vi "CC Script GUI.vi"(10 "Standalone":bool=TRUE, 11 "Cmd Qs":T1) -> ()   [LabVIEW 2024]
uses:
  Subsystems/SS cluster Command Queues.ctl
  Subsystems/SS typedef Cmd Queue Reference.ctl
  Subsystems/SS typedef cluster Instrument Command Queue Data.ctl
  CC cluster Script Panel Defaults.ctl
  typedefs/CC Script Step.ctl
  typedefs/CC enum Script Action.ctl
  typedefs/CC cluster Exposure.ctl
  Detector/Detector Class/Detector enum Detector Integration Mode.ctl
  typedefs/CC cluster Object.ctl
  typedefs/CC cluster sidereal rate.ctl
  typedefs/CC cluster RA and DEC.ctl
  typedefs/cc cluster muRA muDEC.ctl
  Telescope/CC cluster Telescope Offsets.ctl
  typedefs/CC cluster Acquire Parameters.ctl
  Subsystems/SS cluster Script Status Queue.ctl
  typedefs/CC cluster Random Dithering.ctl
  typedefs/CC Dithering.ctl
  typedefs/CC cluster Offset Dithering.ctl
  typedefs/CC Dithering Offsets.ctl
  typedefs/CC cluster Observation Record.ctl
  Subsystems/SS cluster New Image Data.ctl
  hk-channel-class/hk-channel-class/HK Item/HK Item.lvclass
  Subsystems/SS cluster Data Queue type.ctl
  typedefs/CC cluster Observation.ctl
  Observation Queue/CC enum Observation Status.ctl
  typedefs/CC cluster Observation Dither Options.ctl
  typedefs/CC enum Dither Selection.ctl
  typedefs/CC cluster Script.ctl
  typedefs/CC cluster Script Status Data.ctl
  typedefs/CC cluster Pause Parameters.ctl
  Filter Wheel/FW cmd Q Move Parameters.ctl
  Logging/CC enum Current Values Action.ctl
  Focus/Focus cluster MoveFocus Command Parameters.ctl
  CC Rd Wr Script Action.ctl
  3a551b90-7109-44fc-bb48-53d4c8d7d9ea.vi
  fb980131-14b8-4ba4-a5ba-d8795c8df878.vi
  73e8f019-b90d-454d-a375-f578a22e9470.vi
  6180e3d0-9506-4a5f-afbf-da5a1e2ce68c.vi
  79eba822-2b6b-4a1a-8f0f-f154aabb2b36.vi
  hk-channel-class/hk-channel-class/HK Table/HK Table.lvclass
  <vilib>/Utility/Data Type/NI_Data Type.lvlib
panel:
  in  "Script Path":path
  in  "Pause Button":bool
  out "Running":bool
  in  "Close":bool
  in  "Stop Script":bool
  in  "New Script":bool
  in  "Edit Script":bool
  in  "Run Script":bool
  in  "Script":string(combo)
  in  "Script":i32(listbox)
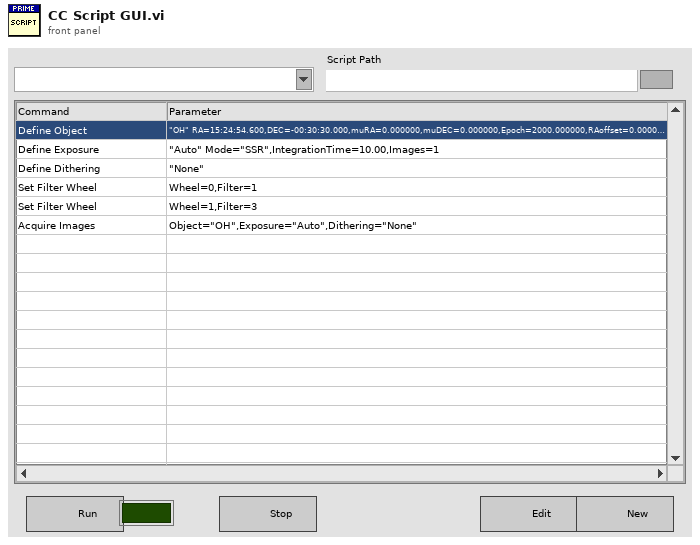
[diagram p1: front panel]
types:
  T1 = typedef "SS cluster Command Queues.ctl" = cluster{"Telescope Q":T2, "Filter Wheel Q":T2, "Script Q":T2, "CryoServer Q":T2, "Detector Q":T2, "Focus Q":T2}
  T2 = typedef "SS typedef Cmd Queue Reference.ctl" = refnum<queue>
  T3 = typedef "CC cluster Script Panel Defaults.ctl" = cluster{"Script Name":string, "Script Path":path}
  T4 = typedef "CC Script Step.ctl" = cluster{"Action":T5, "Data":variant}
  T5 = typedef "CC enum Script Action.ctl" = enum16{"Noop", "Define Object", "Define Exposure", "Define Dithering", "Acquire Images", "Set Filter Wheel", "Telescope Home", "Telescope Move", "Telescope RA DEC", "Focus Move Relative", "Focus Move Absolute", "Focus Set Home", "Macro", "Pause", "Ask User", "Define Random Dither"}
  T6 = typedef "CC cluster Exposure.ctl" = cluster{"Mode":T7, "Integration Time":dbl, "Name":string, "Images":i32}
  T7 = typedef "Detector enum Detector Integration Mode.ctl" = enum16{"SSR", "CDS", "MEAN", "MEDIAN", "MODE", "MIIN", "MAX"}
  T8 = typedef "CC cluster Object.ctl" = cluster{"Object":cluster{"Name":string}, "Sidereal Rate":T9, "RA and DEC":T10, "muRA muDEC Epoch":T11, "Offsets":T12}
  T9 = typedef "CC cluster sidereal rate.ctl" = cluster{"dRA":dbl, "dDEC":dbl}
  T10 = typedef "CC cluster RA and DEC.ctl" = cluster{"RA":dbl, "DEC":dbl}
  T11 = typedef "cc cluster muRA muDEC.ctl" = cluster{"muRA":dbl, "muDEC":dbl, "Epoch":dbl}
  T12 = typedef "CC cluster Telescope Offsets.ctl" = cluster{"RA":dbl, "DEC":dbl, "ROT":dbl}
  T13 = typedef "CC cluster Acquire Parameters.ctl" = cluster{"Object":string, "Exposure":string, "Dithering":string}
  T14 = typedef "CC cluster Random Dithering.ctl" = cluster{"Count":i32, "Radius":dbl, "Name":string}
  T15 = typedef "CC Dithering.ctl" = cluster{"Name":string, "Dithering Offsets":T16}
  T16 = typedef "CC cluster Offset Dithering.ctl" = cluster{"Offsets":T17[]}
  T17 = typedef "CC Dithering Offsets.ctl" = cluster{"DEC":dbl, "RA":dbl}
  T18 = typedef "CC cluster Observation Record.ctl" = cluster{"Start Time":timestamp, "Script":string, "Object":string, "Detector Settings":string, "Dithering Type":string, "Filter":string, "Images":i32}
  T19 = typedef "SS cluster New Image Data.ctl" = cluster{"Frame number":i32, "Detector #":u16, "FITS file":path, "File size":i64}
  T20 = typedef "CC cluster Observation.ctl" = cluster{"Priority":i32, "ID":string, "Observer":string, "Obj Name":string, "Obj Type":string, "RA and DEC String":cluster{"RA":string, "DEC":string}, "Filter Wheel 1":string, "Filter Wheel 2":string, "Integration Time":dbl, "Observation Status":T21, "Offsets":T12, "Images":i32, "Dither Options":T22, "Comment 1":string, "Comment 2":string}
  T21 = typedef "CC enum Observation Status.ctl" = enum16{"Ready", "Running", "Done", "Error"}
  T22 = typedef "CC cluster Observation Dither Options.ctl" = cluster{"Dither":T23, "Dither Radius":dbl, "Dither Points":i32, "Dither Phase":dbl}
  T23 = typedef "CC enum Dither Selection.ctl" = enum16{"None", "Circle", "Random"}
  T24 = cluster{"state":refnum<user-event>, "Script Settings":T3, "Script":T4[], "Cmd Qs":T1, "Parameters":variant, "step":i32, "Script Running":bool, "timer":timestamp, "Script State":string, "Exposure":T6, "Object Map":map{string, T8}, "Acq Settings":T13, "target":T8, "Exp Map":map{string, T6}, "Script Status Q":refnum<queue>, "Images Received":bool, "script edit ref":refnum<vi>, "Run Script":T4[], "Dither":cluster{"Dither Type":bool, "Random Dither":T14, "Offset Dithering":T15, "index":i32}, "Obs List":T18[], "Obs":T18, "images":T19[], "Channel List":refnum<class "HK Item.lvclass">[], "Data Q":refnum<queue>, "Total Images":i32, "paused":bool, "Target RA and DEC":T10, "Image idx":i32, "Observation":T20}
  T25 = enum8{"Enabled", "Disabled", "Disabled and Grayed Out"}
  T26 = typedef "SS typedef cluster Instrument Command Queue Data.ctl" = cluster{"Cmd":string, "Parameters":variant}
  T27 = typedef "SS cluster Data Queue type.ctl" = cluster{"Source":string, "Type":string, "Data":variant}
  T28 = typedef "SS cluster Script Status Queue.ctl" = cluster{"Msg":string, "Data":variant}
  T29 = typedef "CC cluster Script.ctl" = cluster{"Name":string, "Script":T4[]}
  T30 = typedef "CC cluster Script Status Data.ctl" = cluster{"Time":timestamp, "Running":bool, "Step":i32, "Script Name":string, "Step Name":string}
  T31 = typedef "CC cluster Pause Parameters.ctl" = cluster{"Time (s)":dbl}
  T32 = typedef "CC enum Current Values Action.ctl" = enum16{"Init", "Write Item", "Write Array", "Read Item", "Read Array", "Read All", "Add Channels", "New File", "Add Message", "Get Current Values", "Close"}
  T33 = typedef "FW cmd Q Move Parameters.ctl" = cluster{"Wheel ID":i32, "Position":i32}
  T34 = typedef "Focus cluster MoveFocus Command Parameters.ctl" = cluster{"Motor":i32, "Position":i32}
  T35 = typedef "CC Rd Wr Script Action.ctl" = enum16{"Read", "Write", "List", "Delete"}
  T36 = cluster{"Dither Type":bool, "Random Dither":T14, "Offset Dithering":T15, "index":i32}
  T37 = typedef "CC cluster Dithering.ctl" = cluster{"Dither Type":bool, "Random Dither":T14, "Offset Dithering":T15, "index":i32}
  T38 = typedef "LVPoint32TypeDef.ctl" = cluster{"Horizontal":i32, "Vertical":i32}
  T39 = typedef "LVRowAndColumnTypeDef.ctl" = cluster{"Row":i32, "Column":i32}
  T40 = enum32{"Invalid", "Standard", "Closed", "Hidden", "Minimized", "Maximized"}
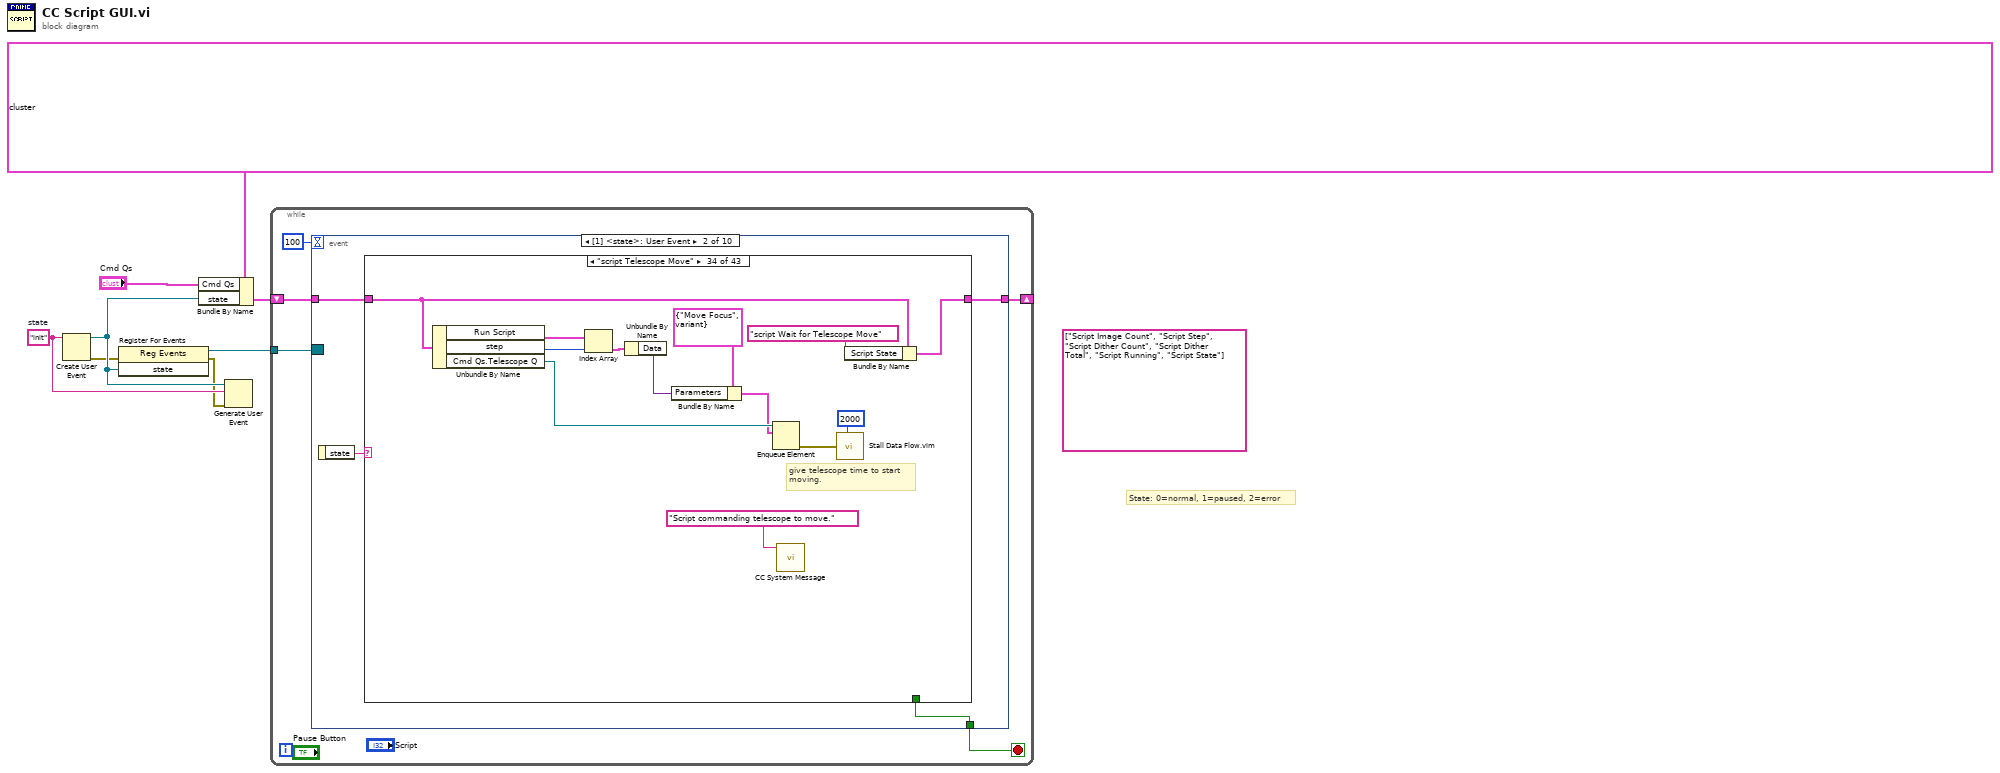
[diagram p0: block diagram]
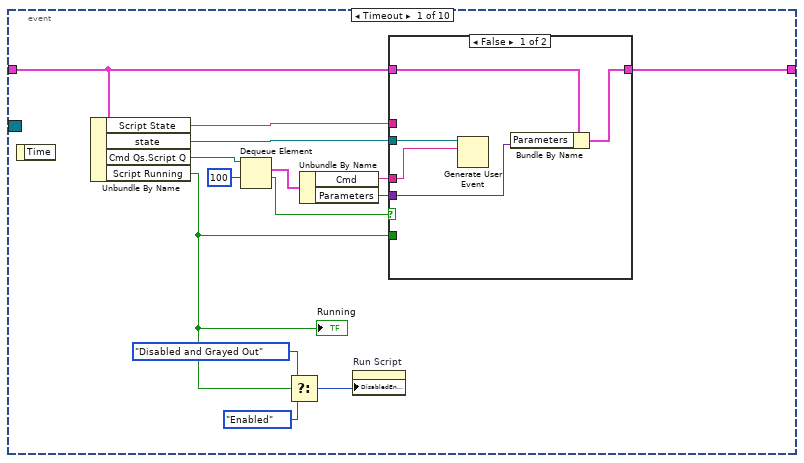
[diagram p2: hidden frame]
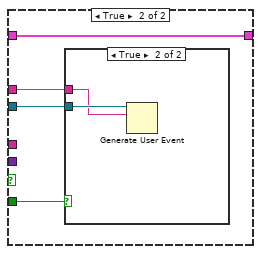
[diagram p3: hidden frame]
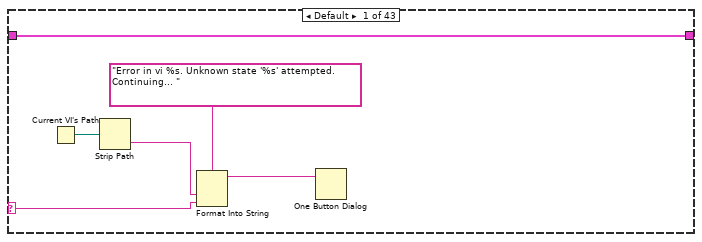
[diagram p5: hidden frame]
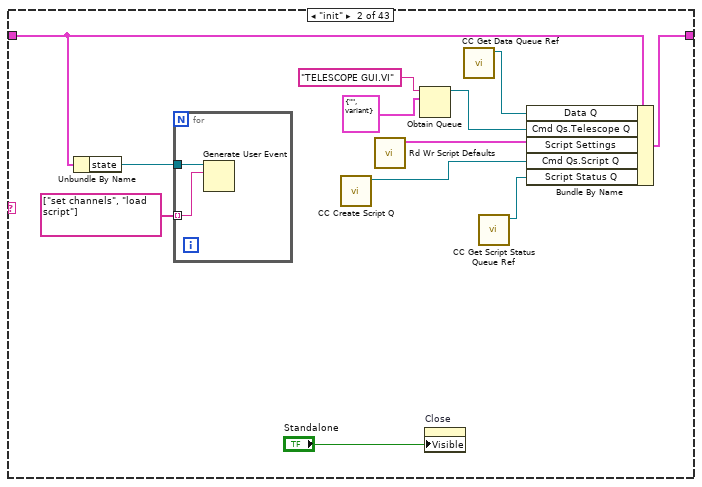
[diagram p6: hidden frame]
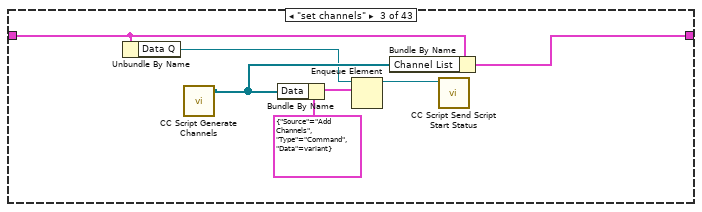
[diagram p7: hidden frame]
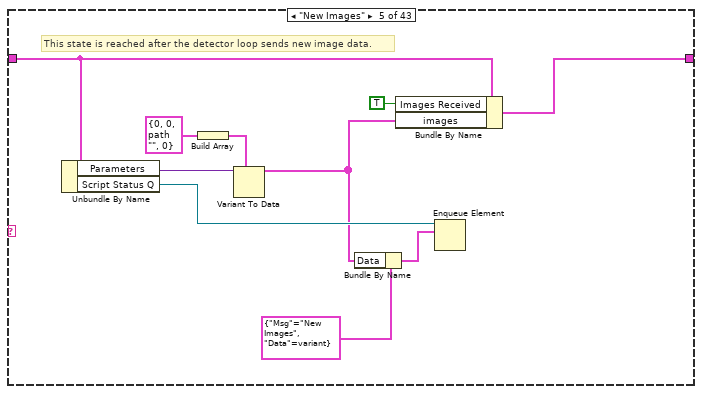
[diagram p9: hidden frame]
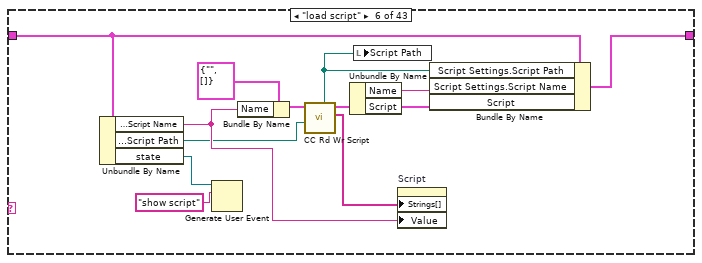
[diagram p10: hidden frame]
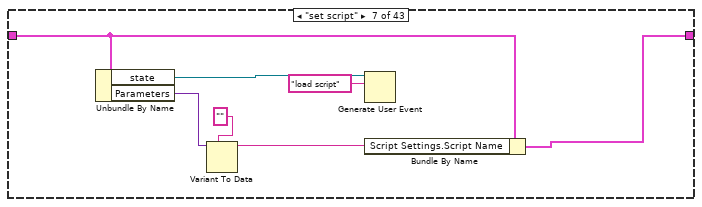
[diagram p11: hidden frame]
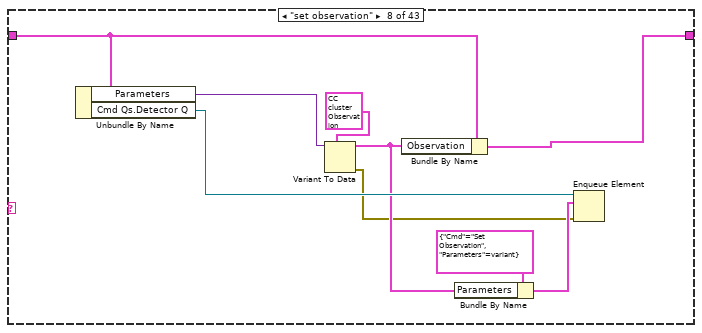
[diagram p12: hidden frame]
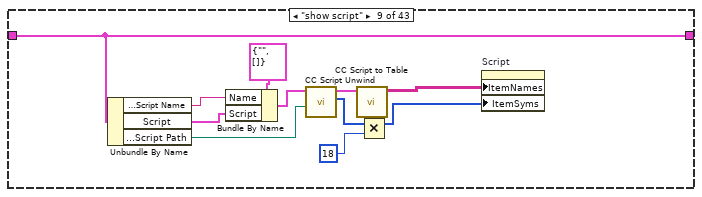
[diagram p13: hidden frame]
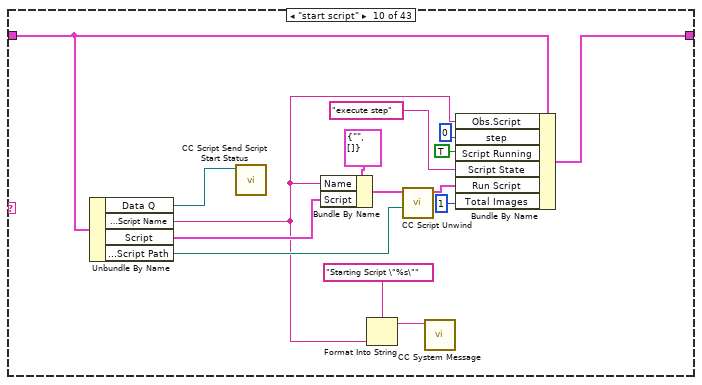
[diagram p14: hidden frame]
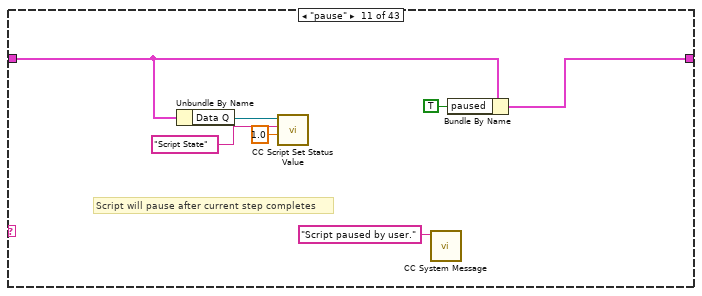
[diagram p15: hidden frame]
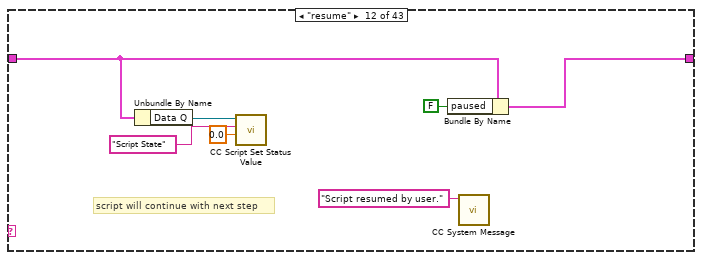
[diagram p16: hidden frame]
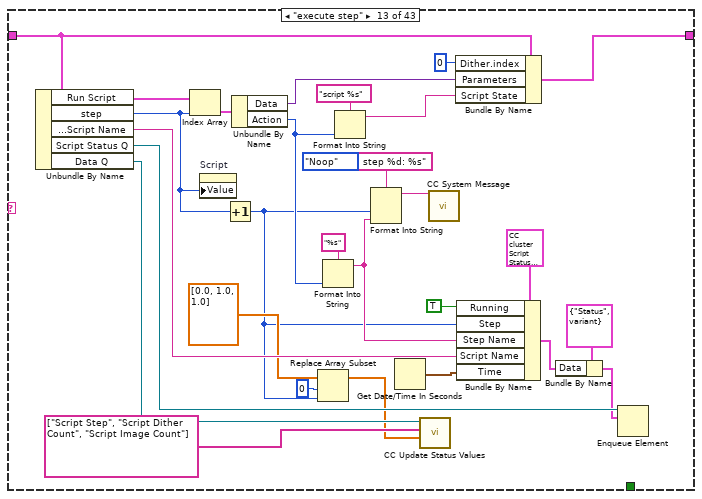
[diagram p17: hidden frame]
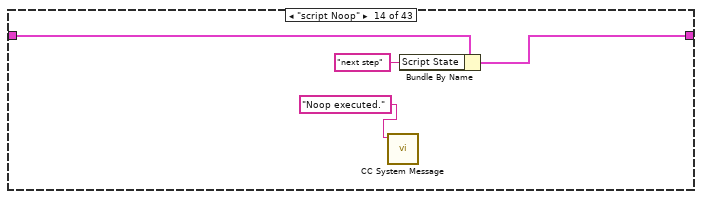
[diagram p18: hidden frame]
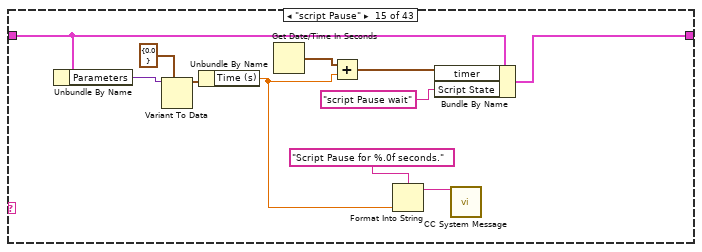
[diagram p19: hidden frame]
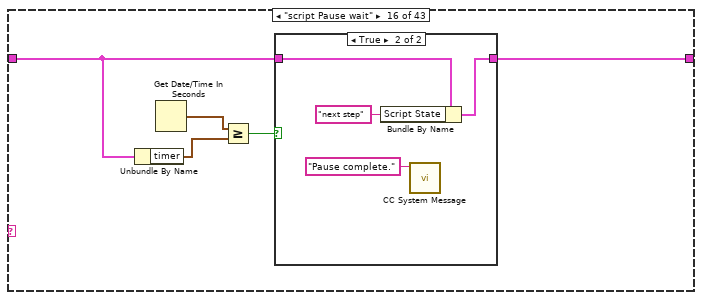
[diagram p20: hidden frame]
diagram:
  (unwired) string[] ["Script Image Count", "Script Step", "Script Dither Count", "Script Dither Total", "Script Running", "Script State"]
  w4 = "init"  # state
  # "State: 0=normal, 1=paused, 2=error"
  n1 = Create User Event(user event datatype=w4) -> (user event=w6:refnum<user-event>, error out=w2:errorcluster)  [unwired: 1 in]
  n2 = register-events(error in=w2, w6) -> (reference out=w5:refnum<event-registration>, error out=w3:errorcluster)  [unwired: 1 in]
  n3 = Bundle By Name(cluster=T24 {"state"=refnum, "Script Settings"={"Script Name"="", "Script Path"=path ""}, "Script"=[], "Cmd Qs"={"Telescope Q"=refnum, "Filter Wheel Q"=refnum, "Script Q"=refnum, "CryoServer Q"=refnum, "Detector Q"=refnum, "Focus Q"=refnum}, "Parameters"=variant, "step"=0, "Script Running"=FALSE, "timer"=timestamp(0 s since 1904-01-01), "Script State"="", "Exposure"={"Mode"=enum."CDS", "Integration Time"=1.0, "Name"="", "Images"=1}, "Object Map"={}, "Acq Settings"={"Object"="", "Exposure"="", "Dithering"=""}, "target"={"Object"={"Name"=""}, "Sidereal Rate"={"dRA"=0.0, "dDEC"=0.0}, "RA and DEC"={"RA"=0.0, "DEC"=0.0}, "muRA muDEC Epoch"={"muRA"=0.0, "muDEC"=0.0, "Epoch"=0.0}, "Offsets"={"RA"=0.0, "DEC"=0.0, "ROT"=0.0}}, "Exp Map"={}, "Script Status Q"=refnum, "Images Received"=FALSE, "script edit ref"=refnum, "Run Script"=[], "Dither"={"Dither Type"=FALSE, "Random Dither"={"Count"=1, "Radius"=1.0, "Name"=""}, "Offset Dithering"={"Name"="", "Dithering Offsets"={"Offsets"=[]}}, "index"=0}, "Obs List"=[], "Obs"={"Start Time"=timestamp(0 s since 1904-01-01), "Script"="", "Object"="", "Detector Settings"="", "Dithering Type"="", "Filter"="", "Images"=0}, "images"=[], "Channel List"=[], "Data Q"=refnum, "Total Images"=0, "paused"=FALSE, "Target RA and DEC"={"RA"=0.0, "DEC"=0.0}, "Image idx"=0, "Observation"={"Priority"=0, "ID"="", "Observer"="", "Obj Name"="", "Obj Type"="", "RA and DEC String"={"RA"="HH:MM:SS.nnn", "DEC"="DEG:arcmin:arcsec.nn"}, "Filter Wheel 1"="", "Filter Wheel 2"="", "Integration Time"=0.0, "Observation Status"=enum."Ready", "Offsets"={"RA"=0.0, "DEC"=0.0, "ROT"=0.0}, "Images"=0, "Dither Options"={"Dither"=enum."None", "Dither Radius"=0.0, "Dither Points"=0, "Dither Phase"=0.0}, "Comment 1"="", "Comment 2"=""}}, "Cmd Qs"="Cmd Qs", "state"=w6) -> (w7:T24)
  n4 = Generate User Event(user event=w6, event data cluster=w4, error in=w3) -> ()  [unwired: 1 in, 2 out]
  n5 = while {
    tunnel: w5 -> [w13]
    shift-right: [w11] -> _
    shift-left: w7 -> [w12]
    stop <- w10 stop-if-true
    n6 = event shown="[1] <state>: User Event" {
      selector: w13 -> [_ _ _ _ _ _ _ _ _ _]
      dyn-events: _ -> [_ _ _ _ _ _ _ _ _ _]
      timeout: 100 -> [_ _ _ _ _ _ _ _ _ _]
      tunnel: w12 -> [w21 w41 w677 w680 w695 w737 w742 w764 w767 w770]
      tunnel: [w19 w40 w674 w680 w694 w738 w743 w764 w767 w770] -> w11
      tunnel: [_ w39 _ _ _ _ _ _ _ _] -> w10
      event Timeout {
        n7 = event-data() -> ()  [unwired: 1 in, 1 out]
        n8 = Unbundle By Name(w21) -> ("Script State"=w18:string, "state"=w22:refnum<user-event>, "Cmd Qs.Script Q"=w27:T2, "Script Running"=w17:bool)
        "Running" <- w17
        n9 = Dequeue Element(queue=w27, timeout in ms (-1)=100) -> (element=w25:T26, timed out?=w24:bool)  [unwired: 1 in, 2 out]
        n10 = Select(t=T25."Disabled and Grayed Out" ("Disabled"), s=w17, f=T25."Enabled" ("Disabled")) -> (s? t:f=w14:T25)
        n11 = Unbundle By Name(w25) -> ("Cmd"=w23:string, "Parameters"=w20:variant)
        n12 = property on="Run Script" class="Bool"("DisabledEnum"=w14) -> ()  [unwired: 2 in, 2 out]
        n13 = case shown="False" w24 {
          tunnel: w23 -> [w31 _]
          tunnel: w22 -> [w32 w34]
          tunnel: w21 -> [w30 w36]
          tunnel: w20 -> [w29 _]
          tunnel: [w28 w36] -> w19
          tunnel: w17 -> [_ w35]
          tunnel: w18 -> [_ w33]
          frame False {
            n14 = Generate User Event(user event=w32, event data cluster=w31) -> ()  [unwired: 2 in, 2 out]
            n15 = Bundle By Name(cluster=w30, "Parameters"=w29) -> (w28:T24)
          }
          frame True {
            n16 = case shown="True" w35 {
              tunnel: w34 -> [_ w38]
              tunnel: w33 -> [_ w37]
              frame False {
              }
              frame True {
                n17 = Generate User Event(user event=w38, event data cluster=w37) -> ()  [unwired: 2 in, 2 out]
              }
            }
          }
        }
      }
      event User Event {
        n18 = event-data() -> ("state"=w42:string)  [unwired: 1 in]
        n19 = case shown="\"script Telescope Move\"" w42 {
          selector: w42 -> [w47 _ _ _ _ _ _ _ _ _ _ _ _ _ _ _ _ _ _ _ _ _ _ w314 _ _ _ _ _ _ w465 _ _ _ _ _ _ _ _ _ _ _ _]
          tunnel: w41 -> [w43 w58 w65 w70 w75 w84 w95 w107 w120 w134 w137 w147 w169 w178 w183 w194 w207 w228 w240 w255 w270 w289 w310 w316 w337 w347 w357 w379 w404 w451 w462 w494 w519 w543 w556 w575 w584 w599 w615 w643 w651 w662 w670]
          tunnel: [w43 w59 w66 w70 w76 w85 w96 w108 w120 w135 w141 w148 w170 w179 w184 w193 w210 w229 w243 w258 w273 w291 w312 w317 w339 w349 w359 w380 w407 w452 w463 w496 w517 w544 w557 w576 w585 w600 w613 w644 w652 w666 w670] -> w40
          tunnel: [_ _ _ _ _ _ _ _ _ _ _ _ _ _ _ _ _ _ _ _ _ _ _ _ _ _ _ _ _ _ _ _ _ _ _ _ _ _ _ _ _ _ TRUE] -> w39
          frame Default {
            n20 = Current VI's Path() -> (path=w46:path)
            n21 = Strip Path(path=w46) -> (name=w45:string)  [unwired: 1 out]
            n22 = Format Into String(format string="Error in vi %s. Unknown state '%s' attempted. Continuing... ", w45, w47) -> (resulting string=w44:string)  [unwired: 2 in, 1 out]
            n23 = One Button Dialog(message=w44) -> ()  [unwired: 1 in, 1 out]
          }
          frame "init" {
            n24 = Unbundle By Name(w58) -> ("state"=w57:refnum<user-event>)
            n25 = for {
              tunnel: w57 -> [w62]
              tunnel: string[] ["set channels", "load script"] -> [w61] mode=indexing
              n26 = Generate User Event(user event=w62, event data cluster=w61) -> ()  [unwired: 2 in, 2 out]
            }
            n27 = call "CC Create Script Q.vi"() -> ("Script Q"=w49:refnum<queue>)  [unwired: 10 in, 1 out]
            n28 = call "Rd Wr Script Defaults.vi"() -> ("Script Settings"=w60:T3)  [unwired: 10 in, 1 out]
            n29 = Obtain Queue(name (unnamed)="TELESCOPE GUI.VI", element data type=T26 {"Cmd"="", "Parameters"=variant}) -> (queue out=w52:refnum<queue>)  [unwired: 3 in, 2 out]
            n30 = property on="Close" class="Bool"("Visible"="Standalone") -> ()  [unwired: 2 in, 2 out]
            n31 = call "CC Get Data Queue Ref.vi"() -> ("Data Q"=w50:refnum<queue>)  [unwired: 10 in, 1 out]
            n32 = call "CC Get Script Status Queue Ref.vi"() -> ("Script Status Q"=w55:refnum<queue>)  [unwired: 10 in, 1 out]
            n33 = Bundle By Name(cluster=w58, "Data Q"=w50, "Cmd Qs.Telescope Q"=w52, "Script Settings"=w60, "Cmd Qs.Script Q"=w49, "Script Status Q"=w55) -> (w59:T24)
          }
          frame "set channels" {
            n34 = Unbundle By Name(w65) -> ("Data Q"=w64:refnum<queue>)
            n35 = call "CC Script Generate Channels.vi"() -> ("Channel List"=w67:refnum<class "HK Item.lvclass">[])  [unwired: 9 in, 2 out]
            n36 = Bundle By Name(cluster=T27 {"Source"="Add Channels", "Type"="Command", "Data"=variant} ("element"), "Data"=w67) -> (w69:T27)
            n37 = Enqueue Element(queue=w64, element=w69) -> (queue out=w63:refnum<queue>)  [unwired: 2 in, 2 out]
            n38 = Bundle By Name(cluster=w65, "Channel List"=w67) -> (w66:T24)
            n39 = call "CC Script Send Script Start Status.vi"("Data Q"=w63) -> ()  [unwired: 10 in, 1 out]
          }
          frame "idle" {
          }
          frame "New Images" {
            # "This state is reached after the detector loop sends new image data."
            n40 = Unbundle By Name(w75) -> ("Parameters"=w79:variant, "Script Status Q"=w74:refnum<queue>)
            n41 = Build Array(T19 {"Frame number"=0, "Detector #"=0, "FITS file"=path "", "File size"=0} ("New Image")) -> (w78:T19[])
            n42 = Variant To Data(type=w78, Variant=w79) -> (data=w71:T19[])  [unwired: 1 in, 1 out]
            n43 = Bundle By Name(cluster=T28 {"Msg"="New Images", "Data"=variant} ("element"), "Data"=w71) -> (w72:T28)
            n44 = Bundle By Name(cluster=w75, "Images Received"=TRUE, "images"=w71) -> (w76:T24)
            n45 = Enqueue Element(queue=w74, element=w72) -> ()  [unwired: 2 in, 3 out]
          }
          frame "load script" {
            n46 = Unbundle By Name(w84) -> ("Script Settings.Script Name"=w83:string, "Script Settings.Script Path"=w82:path, "state"=w88:refnum<user-event>)
            n47 = Generate User Event(user event=w88, event data cluster="show script" ("event data")) -> ()  [unwired: 2 in, 2 out]
            n48 = Bundle By Name(cluster=T29 {"Name"="", "Script"=[]} ("Script"), "Name"=w83) -> (w93:T29)
            n49 = call "CC Rd Wr Script.vi"("Script Path"=w82, "Script"=w93) -> ("Script List"=w91:string[], "Script"=w92:T29, "Script Path"=w81:path)  [unwired: 4 in, 3 out]
            n50 = Unbundle By Name(w92) -> ("Name"=w86:string, "Script"=w87:T4[])
            n51 = local write "Script Path"(w81) -> ()
            n52 = property on="Script" class="CmbBox"("Strings[]"=w91, "Value"=w83) -> ()  [unwired: 2 in, 2 out]
            n53 = Bundle By Name(cluster=w84, "Script Settings.Script Path"=w81, "Script Settings.Script Name"=w86, "Script"=w87) -> (w85:T24)
          }
          frame "set script" {
            n54 = Unbundle By Name(w95) -> ("state"=w98:refnum<user-event>, "Parameters"=w100:variant)
            n55 = Variant To Data(type="", Variant=w100) -> (data=w97:string)  [unwired: 1 in, 1 out]
            n56 = Generate User Event(user event=w98, event data cluster="load script" ("event data")) -> ()  [unwired: 2 in, 2 out]
            n57 = Bundle By Name(cluster=w95, "Script Settings.Script Name"=w97) -> (w96:T24)
          }
          frame "set observation" {
            n58 = Unbundle By Name(w107) -> ("Parameters"=w109:variant, "Cmd Qs.Detector Q"=w105:T2)
            n59 = Variant To Data(type=T20 {"Priority"=0, "ID"="", "Observer"="", "Obj Name"="", "Obj Type"="", "RA and DEC String"={"RA"="HH:MM:SS.nnn", "DEC"="DEG:arcmin:arcsec.nn"}, "Filter Wheel 1"="", "Filter Wheel 2"="", "Integration Time"=0.0, "Observation Status"=enum."Error", "Offsets"={"RA"=0.0, "DEC"=0.0, "ROT"=0.0}, "Images"=0, "Dither Options"={"Dither"=enum."None", "Dither Radius"=0.0, "Dither Points"=0, "Dither Phase"=0.0}, "Comment 1"="", "Comment 2"=""} ("element"), Variant=w109) -> (data=w102:T20, error out=w101:errorcluster)  [unwired: 1 in]
            n60 = Bundle By Name(cluster=w107, "Observation"=w102) -> (w108:T24)
            n61 = Bundle By Name(cluster=T26 {"Cmd"="Set Observation", "Parameters"=variant} ("element"), "Parameters"=w102) -> (w103:T26)
            n62 = Enqueue Element(queue=w105, element=w103, error in (no error)=w101) -> ()  [unwired: 1 in, 3 out]
          }
          frame "show script" {
            n63 = Unbundle By Name(w120) -> ("Script Settings.Script Name"=w117:string, "Script"=w116:T4[], "Script Settings.Script Path"=w110:path)
            n64 = Bundle By Name(cluster=T29 {"Name"="", "Script"=[]} ("Script"), "Name"=w117, "Script"=w116) -> (w115:T29)
            n65 = call "CC Script Unwind.vi"("Script Path"=w110, "Script"=w115) -> ("Indent"=w113:i32[], "Unwound Script"=w114:T4[])  [unwired: 7 in, 1 out]
            n66 = call "CC Script to Table.vi"("Script"=w114) -> ("table"=w119:string[][])  [unwired: 9 in, 1 out]
            n67 = Multiply(x=w113, y=18) -> (x*y=w112:i32[])
            n68 = property on="Script" class="MCListbox (strict)"("ItemNames"=w119, "ItemSyms"=w112) -> ()  [unwired: 2 in, 2 out]
          }
          frame "start script" {
            n69 = Unbundle By Name(w134) -> ("Data Q"=w122:refnum<queue>, "Script Settings.Script Name"=w123:string, "Script"=w127:T4[], "Script Settings.Script Path"=w124:path)
            n70 = call "CC Script Send Script Start Status.vi"("Data Q"=w122) -> ()  [unwired: 10 in, 1 out]
            n71 = Bundle By Name(cluster=T29 {"Name"="", "Script"=[]} ("Script"), "Name"=w123, "Script"=w127) -> (w126:T29)
            n72 = Format Into String(format string="Starting Script \"%s\"" ("Message"), w123) -> (resulting string=w131:string)  [unwired: 2 in, 1 out]
            n73 = call "CC Script Unwind.vi"("Script Path"=w124, "Script"=w126) -> ("Unwound Script"=w125:T4[])  [unwired: 7 in, 2 out]
            n74 = call "CC System Message.vi"("Message"=w131) -> ()  [unwired: 10 in, 1 out]
            n75 = Bundle By Name(cluster=w134, "Obs.Script"=w123, "step"=0, "Script Running"=TRUE, "Script State"="execute step" ("event data"), "Run Script"=w125, "Total Images"=1 ("Image Count")) -> (w135:T24)
          }
          frame "pause" {
            # "Script will pause after current step completes"
            n76 = Unbundle By Name(w137) -> ("Data Q"=w140:refnum<queue>)
            n77 = call "CC Script Set Status Value.vi"("Value"=1.0, "Ch Name"="Script State", "Data Q"=w140) -> ()  [unwired: 8 in, 1 out]
            n78 = call "CC System Message.vi"("Message"="Script paused by user.") -> ()  [unwired: 10 in, 1 out]
            n79 = Bundle By Name(cluster=w137, "paused"=TRUE) -> (w141:T24)
          }
          frame "resume" {
            # "script will continue with next step"
            n80 = Unbundle By Name(w147) -> ("Data Q"=w146:refnum<queue>)
            n81 = call "CC Script Set Status Value.vi"("Value"=0.0, "Ch Name"="Script State", "Data Q"=w146) -> ()  [unwired: 8 in, 1 out]
            n82 = Bundle By Name(cluster=w147, "paused"=FALSE) -> (w148:T24)
            n83 = call "CC System Message.vi"("Message"="Script resumed by user.") -> ()  [unwired: 10 in, 1 out]
          }
          frame "execute step" {
            (unwired) CC_enum_Script_Action."Noop" ("Action")
            n84 = Unbundle By Name(w169) -> ("Run Script"=w177:T4[], "step"=w173:i32, "Script Settings.Script Name"=w162:string, "Script Status Q"=w160:refnum<queue>, "Data Q"=w155:refnum<queue>)
            n85 = Index Array(array=w177, index=w173) -> (element=w176:T4)
            n86 = property on="Script" class="MCListbox (strict)"("Value"=w173) -> ()  [unwired: 2 in, 2 out]
            n87 = Increment(x=w173) -> (x+1=w151:i32)
            n88 = Unbundle By Name(w176) -> ("Data"=w168:variant, "Action"=w164:T5)
            n89 = Replace Array Subset(array=dbl[] [0.0, 1.0, 1.0] ("Values"), new element=w151, index=0) -> (w150:dbl[])
            n90 = Format Into String(format string="%s", w164) -> (resulting string=w163:string)  [unwired: 2 in, 1 out]
            n91 = Format Into String(format string="script %s", w164) -> (resulting string=w171:string)  [unwired: 2 in, 1 out]
            n92 = Format Into String(format string="Executing step %d: %s", w151, w163) -> (resulting string=w172:string)  [unwired: 2 in, 1 out]
            n93 = Get Date/Time In Seconds() -> (seconds since 1Jan1904=w161:timestamp)
            n94 = call "CC Update Status Values.vi"("Values"=w150, "names"=string[] ["Script Step", "Script Dither Count", "Script Image Count"], "Data Q"=w155) -> ()  [unwired: 8 in, 1 out]
            n95 = call "CC System Message.vi"("Message"=w172) -> ()  [unwired: 10 in, 1 out]
            n96 = Bundle By Name(cluster=w169, "Dither.index"=0, "Parameters"=w168, "Script State"=w171) -> (w170:T24)
            n97 = Bundle By Name(cluster=T30 {"Time"=timestamp(0 s since 1904-01-01), "Running"=FALSE, "Step"=0, "Script Name"="", "Step Name"=""}, "Running"=TRUE, "Step"=w151, "Step Name"=w163, "Script Name"=w162, "Time"=w161) -> (w158:T30)
            n98 = Bundle By Name(cluster=T28 {"Msg"="Status", "Data"=variant} ("element"), "Data"=w158) -> (w157:T28)
            n99 = Enqueue Element(queue=w160, element=w157) -> ()  [unwired: 2 in, 3 out]
          }
          frame "script Noop" {
            n100 = call "CC System Message.vi"("Message"="Noop executed." ("format string")) -> ()  [unwired: 10 in, 1 out]
            n101 = Bundle By Name(cluster=w178, "Script State"="next step" ("event data")) -> (w179:T24)
          }
          frame "script Pause" {
            n102 = Unbundle By Name(w183) -> ("Parameters"=w190:variant)
            n103 = Variant To Data(type=T31 {"Time (s)"=0.0} ("Pause Parameters"), Variant=w190) -> (data=w188:T31)  [unwired: 1 in, 1 out]
            n104 = Unbundle By Name(w188) -> ("Time (s)"=w186:dbl)
            n105 = Get Date/Time In Seconds() -> (seconds since 1Jan1904=w187:timestamp)
            n106 = Add(x=w187, y=w186) -> (x+y=w185:timestamp)
            n107 = Format Into String(format string="Script Pause for %.0f seconds.", w186) -> (resulting string=w191:string)  [unwired: 2 in, 1 out]
            n108 = Bundle By Name(cluster=w183, "timer"=w185, "Script State"="script Pause wait" ("event data")) -> (w184:T24)
            n109 = call "CC System Message.vi"("Message"=w191) -> ()  [unwired: 10 in, 1 out]
          }
          frame "script Pause wait" {
            n110 = Unbundle By Name(w194) -> ("timer"=w196:timestamp)
            n111 = Get Date/Time In Seconds() -> (seconds since 1Jan1904=w197:timestamp)
            n112 = Greater Or Equal?(x=w197, y=w196) -> (x >= y?=w195:bool)
            n113 = case shown="True" w195 {
              tunnel: w194 -> [w198 w202]
              tunnel: [w198 w200] -> w193
              frame False {
              }
              frame True {
                n114 = Bundle By Name(cluster=w202, "Script State"="next step") -> (w200:T24)
                n115 = call "CC System Message.vi"("Message"="Pause complete.") -> ()  [unwired: 10 in, 1 out]
              }
            }
          }
          frame "script Macro" {
            n116 = Unbundle By Name(w207) -> ("Parameters"=w208:variant)
            n117 = Variant To Data(type="", Variant=w208) -> (data=w204:string)  [unwired: 1 in, 1 out]
            n118 = Format Into String(format string="Executing Macro %s" ("Message"), w204) -> (resulting string=w203:string)  [unwired: 2 in, 1 out]
            n119 = Bundle By Name(cluster=w207, "Script State"="next step") -> (w210:T24)
            n120 = call "CC System Message.vi"("Message"=w203) -> ()  [unwired: 10 in, 1 out]
          }
          frame "script Define Object" {
            # "Move telescope"
            n121 = Unbundle By Name(w228) -> ("Parameters"=w227:variant, "Object Map"=w225:map{string, T8}, "Cmd Qs.Telescope Q"=w212:T2)
            n122 = Variant To Data(type=T8 {"Object"={"Name"=""}, "Sidereal Rate"={"dRA"=0.0, "dDEC"=0.0}, "RA and DEC"={"RA"=0.0, "DEC"=0.0}, "muRA muDEC Epoch"={"muRA"=0.0, "muDEC"=0.0, "Epoch"=0.0}, "Offsets"={"RA"=0.0, "DEC"=0.0, "ROT"=0.0}} ("Object"), Variant=w227) -> (data=w211:T8)  [unwired: 1 in, 1 out]
            n123 = Unbundle By Name(w211) -> ("Object.Name"=w224:string)
            n124 = Unbundle By Name(w211) -> ("Object.Name"=w221:string, "RA and DEC.RA"=w220:dbl, "RA and DEC.DEC"=w219:dbl, "Offsets.RA"=w217:dbl, "Offsets.DEC"=w216:dbl, "Offsets.ROT"=w215:dbl)
            n125 = Insert Into Map(map in=w225, key=w224, value=w211) -> (map out=w223:map{string, T8})  [unwired: 2 out]
            n126 = Bundle By Name(cluster=w228, "Script State"="next step", "Object Map"=w223) -> (w229:T24)
            n127 = Bundle By Name(cluster=T26 {"Cmd"="Move", "Parameters"=variant} ("element"), "Parameters"=w211) -> (w213:T26)
            n128 = Format Into String(format string="Script defined target object \"%s\" at RA=%f, DEC=%f and RAoffset=%.1f, DECoffset=%.1f, ROToffset=%.1g", w221, w220, w219, w217, w216, w215) -> (resulting string=w218:string)  [unwired: 2 in, 1 out]
            n129 = Enqueue Element(queue=w212, element=w213) -> ()  [unwired: 2 in, 3 out]
            n130 = call "CC System Message.vi"("Message"=w218) -> ()  [unwired: 10 in, 1 out]
          }
          frame "script Define Exposure" {
            n131 = Unbundle By Name(w240) -> ("Exp Map"=w239:map{string, T6}, "Parameters"=w242:variant)
            n132 = Variant To Data(type=T6 {"Mode"=enum."CDS", "Integration Time"=1.0, "Name"="", "Images"=1} ("Exposure"), Variant=w242) -> (data=w237:T6)  [unwired: 1 in, 1 out]
            n133 = Unbundle By Name(w237) -> ("Images"=w231:i32, "Name"=w234:string, "Mode"=w233:T7, "Integration Time"=w232:dbl)
            n134 = Insert Into Map(map in=w239, key=w234, value=w237) -> (map out=w238:map{string, T6})  [unwired: 2 out]
            n135 = Bundle By Name(cluster=w240, "Script State"="next step", "Exp Map"=w238, "Image idx"=w231) -> (w243:T24)
            n136 = Format Into String(format string="Script defined exposure settings \"%s\" mode %s, integration time %f, collection %d images.", w234, w233, w232, w231) -> (resulting string=w235:string)  [unwired: 2 in, 1 out]
            n137 = call "CC System Message.vi"("Message"=w235) -> ()  [unwired: 10 in, 1 out]
          }
          frame "script Define Random Dither" {
            n138 = Unbundle By Name(w255) -> ("Parameters"=w257:variant, "Data Q"=w248:refnum<queue>)
            n139 = Variant To Data(type=T14 {"Count"=1, "Radius"=1.0, "Name"=""} ("Dithering Offsets"), Variant=w257) -> (data=w251:T14)  [unwired: 1 in, 1 out]
            n140 = Unbundle By Name(w251) -> ("Name"=w250:string, "Count"=w246:i32, "Radius"=w249:dbl)
            n141 = Increment(x=w246) -> (x+1=w245:i32)
            n142 = Bundle By Name(cluster=w255, "Script State"="next step", "Dither.Random Dither"=w251, "Dither.Dither Type"=TRUE) -> (w258:T24)
            n143 = Format Into String(format string="Script defined random dithering \"%s\" at %d spots with radius %f", w250, w246, w249) -> (resulting string=w252:string)  [unwired: 2 in, 1 out]
            n144 = call "CC Script Set Status Value.vi"("Value"=w245, "Ch Name"="Script Dither Total", "Data Q"=w248) -> ()  [unwired: 8 in, 1 out]
            n145 = call "CC System Message.vi"("Message"=w252) -> ()  [unwired: 10 in, 1 out]
          }
          frame "script Define Dithering" {
            n146 = Unbundle By Name(w270) -> ("Parameters"=w272:variant, "Data Q"=w262:refnum<queue>)
            n147 = Variant To Data(type=T15 {"Name"="", "Dithering Offsets"={"Offsets"=[]}} ("Dithering Offsets"), Variant=w272) -> (data=w266:T15)  [unwired: 1 in, 1 out]
            n148 = Unbundle By Name(w266) -> ("Name"=w265:string, "Dithering Offsets.Offsets"=w264:T17[])
            n149 = Bundle By Name(cluster=w270, "Script State"="next step", "Dither.Offset Dithering"=w266, "Dither.Dither Type"=FALSE) -> (w273:T24)
            n150 = Array Size(array=w264) -> (size(s)=w261:i32)
            n151 = Increment(x=w261) -> (x+1=w260:i32)
            n152 = Format Into String(format string="Script defined dithering \"%s\" containing %d offsets.", w265, w261) -> (resulting string=w267:string)  [unwired: 2 in, 1 out]
            n153 = call "CC Script Set Status Value.vi"("Value"=w260, "Ch Name"="Script Dither Total", "Data Q"=w262) -> ()  [unwired: 8 in, 1 out]
            n154 = call "CC System Message.vi"("Message"=w267) -> ()  [unwired: 10 in, 1 out]
          }
          frame "script Set Filter Wheel" {
            n155 = Unbundle By Name(w289) -> ("Parameters"=w290:variant)
            n156 = call "CC Log Object.vi"("Action"=CC_enum_Current_Values_Action."Get Current Values") -> ("HK Channel out"=w286:refnum<class "HK Table.lvclass">)  [unwired: 8 in, 2 out]
            n157 = for {
              N: 2 -> [_]
              tunnel: w286 -> [w297]
              tunnel: [w296] -> w282 mode=indexing
              tunnel: "Wheel%d Encoder Position" -> [w295]
              i -> [w294]
              n158 = Format Into String(format string=w295, w294) -> (resulting string=w293:string)  [unwired: 2 in, 1 out]
              n159 = call-dynamic "HK Read Value.vi"("Channel Name"=w293, "HK Channel in"=w297) -> ("Value"=w296:dbl)  [unwired: 4 in, 5 out]
            }
            n160 = Variant To Data(type=T33 {"Wheel ID"=0, "Position"=0}, Variant=w290) -> (data=w287:T33)  [unwired: 1 in, 1 out]
            n161 = Unbundle By Name(w287) -> ("Wheel ID"=w281:i32, "Position"=w279:i32)
            n162 = Index Array(array=w282, index=w281) -> (element=w280:dbl)
            n163 = Equal?(x=w280, y=w279) -> (x = y?=w275:bool)
            n164 = case shown="True" w275 {
              frame False {
              }
              frame True {
                n165 = call "CC System Message.vi"("Message"="Filter already in position.") -> ()  [unwired: 10 in, 1 out]
              }
            }
            n166 = Select(t="next step", s=w275, f="script Filter Wheel Move" ("Script State")) -> (s? t:f=w276:string)
            n167 = Bundle By Name(cluster=w289, "Script State"=w276) -> (w291:T24)
          }
          frame "script Filter Wheel Move" {
            n168 = Unbundle By Name(w310) -> ("Parameters"=w311:variant, "Cmd Qs.Filter Wheel Q"=w309:T2)
            n169 = Variant To Data(type=T33 {"Wheel ID"=0, "Position"=0}, Variant=w311) -> (data=w300:T33, error out=w306:errorcluster)  [unwired: 1 in]
            n170 = Bundle By Name(cluster=T26 {"Cmd"="Move", "Parameters"=variant} ("element"), "Parameters"=w300) -> (w301:T26)
            n171 = Enqueue Element(queue=w309, element=w301, error in (no error)=w306) -> (error out=w305:errorcluster)  [unwired: 1 in, 2 out]
            n172 = Unbundle By Name(w300) -> ("Wheel ID"=w299:i32, "Position"=w298:i32)
            n173 = call "Stall Data Flow.vim"("value in"=w305, "milliseconds to wait"=u32 5000) -> ()  [unwired: 2 out]
            n174 = Format Into String(format string="Script moving filter wheel %d to position %d", w299, w298) -> (resulting string=w302:string)  [unwired: 2 in, 1 out]
            n175 = Bundle By Name(cluster=w310, "Script State"="script Filter Wheel Wait") -> (w312:T24)
            n176 = call "CC System Message.vi"("Message"=w302) -> ()  [unwired: 10 in, 1 out]
          }
          frame "script Filter Wheel Wait" {
            n177 = call "CC Log Object.vi"("Action"=CC_enum_Current_Values_Action."Get Current Values") -> ("HK Channel out"=w324:refnum<class "HK Table.lvclass">)  [unwired: 8 in, 2 out]
            n178 = for {
              N: 2 -> [_]
              tunnel: w324 -> [w330]
              tunnel: [w329] -> w321 mode=indexing
              tunnel: "Wheel%d Moving" -> [w328]
              i -> [w327]
              n179 = Format Into String(format string=w328, w327) -> (resulting string=w326:string)  [unwired: 2 in, 1 out]
              n180 = call-dynamic "HK Read Value.vi"("Channel Name"=w326, "HK Channel in"=w330) -> ("Value"=w329:dbl)  [unwired: 4 in, 5 out]
            }
            n181 = Equal To 0?(x=w321) -> (x = 0?=w320:bool[])
            n182 = And Array Elements(Boolean array=w320) -> (logical AND=w319:bool)
            n183 = Select(t="next step", s=w319, f=w314) -> (s? t:f=w318:string)
            n184 = Bundle By Name(cluster=w316, "Script State"=w318) -> (w317:T24)
          }
          frame "script Focus Move Relative" {
            n185 = Unbundle By Name(w337) -> ("Parameters"=w338:variant, "Cmd Qs.Focus Q"=w336:T2)
            n186 = Variant To Data(type=T34 {"Motor"=0, "Position"=0} ("Cluster"), Variant=w338) -> (data=w334:T34, error out=w333:errorcluster)  [unwired: 1 in]
            n187 = Bundle By Name(cluster=T26 {"Cmd"="FocusMoveRelative", "Parameters"=variant} ("element"), "Parameters"=w334) -> (w332:T26)
            n188 = Enqueue Element(queue=w336, element=w332, error in (no error)=w333) -> ()  [unwired: 1 in, 3 out]
            n189 = Bundle By Name(cluster=w337, "Script State"="next step") -> (w339:T24)
          }
          frame "script Focus Move Absolute" {
            n190 = Unbundle By Name(w347) -> ("Parameters"=w348:variant, "Cmd Qs.Focus Q"=w346:T2)
            n191 = Variant To Data(type=T34 {"Motor"=0, "Position"=0} ("Cluster"), Variant=w348) -> (data=w344:T34, error out=w343:errorcluster)  [unwired: 1 in]
            n192 = Bundle By Name(cluster=T26 {"Cmd"="FocusMoveAbsolute", "Parameters"=variant} ("element"), "Parameters"=w344) -> (w342:T26)
            n193 = Enqueue Element(queue=w346, element=w342, error in (no error)=w343) -> ()  [unwired: 1 in, 3 out]
            n194 = Bundle By Name(cluster=w347, "Script State"="next step") -> (w349:T24)
          }
          frame "script Focus Set Home" {
            n195 = Unbundle By Name(w357) -> ("Parameters"=w358:variant, "Cmd Qs.Focus Q"=w356:T2)
            n196 = Variant To Data(type=0, Variant=w358) -> (data=w354:i32, error out=w353:errorcluster)  [unwired: 1 in]
            n197 = Bundle By Name(cluster=T26 {"Cmd"="FocusSetHome", "Parameters"=variant} ("element"), "Parameters"=w354) -> (w352:T26)
            n198 = Enqueue Element(queue=w356, element=w352, error in (no error)=w353) -> ()  [unwired: 1 in, 3 out]
            n199 = Bundle By Name(cluster=w357, "Script State"="next step") -> (w359:T24)
          }
          frame "script Acquire Images" {
            # "Tell the telescope to move to target."
            n200 = Unbundle By Name(w379) -> ("Exp Map"=w363:map{string, T6}, "Object Map"=w378:map{string, T8}, "Parameters"=w383:variant, "Cmd Qs.Telescope Q"=w381:T2, "Data Q"=w369:refnum<queue>)
            n201 = Variant To Data(type=T13 {"Object"="", "Exposure"="", "Dithering"=""} ("Acquire Parameters"), Variant=w383) -> (data=w364:T13)  [unwired: 1 in, 1 out]
            n202 = Unbundle By Name(w364) -> ("Exposure"=w362:string)
            n203 = Unbundle By Name(w364) -> ("Object"=w370:string)
            n204 = call "CC Script Set Status Value.vi"("Value"=1.0, "Ch Name"="Script Dither Count", "Data Q"=w369) -> ()  [unwired: 8 in, 1 out]
            n205 = Remove From Map(10:w362, 11:w363) -> (1:w361:T6)  [unwired: 2 out]
            n206 = Remove From Map(10:w370, 11:w378) -> (1:w377:T8, 2:w376:bool)  [unwired: 1 out]
            n207 = case shown="False" w376 {
              tunnel: w381 -> [w386 _]
              tunnel: w377 -> [w384 w391]
              tunnel: ["script Acquire Wait Move" ("Script State") "abort script" ("Script State")] -> w375
              tunnel: w370 -> [_ w393]
              tunnel: [w384 w391] -> w366
              frame False {
                n208 = disable-structure shown="Enabled" {
                  disable-tunnel: w386 -> [w390 _]
                  disable-tunnel: w384 -> [w387 _]
                  frame Disabled {
                    n209 = Bundle By Name(cluster=T26 {"Cmd"="Move", "Parameters"=variant} ("element"), "Parameters"=w387) -> (w388:T26)
                    n210 = Enqueue Element(queue=w390, element=w388) -> ()  [unwired: 2 in, 3 out]
                  }
                  frame Enabled {
                    # "Telescope move command\nnow in the Define Object\nstep to save time."
                  }
                }
              }
              frame True {
                n211 = Format Into String(format string="Acquire Images command referred to undefined object \"%s\".", w393) -> (resulting string=w392:string)  [unwired: 2 in, 1 out]
                n212 = call "CC System Message.vi"("Message"=w392) -> ()  [unwired: 10 in, 1 out]
                n213 = One Button Dialog(message=w392) -> ()  [unwired: 1 in, 1 out]
              }
            }
            n214 = Unbundle By Name(w366) -> ("RA and DEC"=w365:T10)
            n215 = Format Into String(format string="Waiting for telescope to target %s", w370) -> (resulting string=w371:string)  [unwired: 2 in, 1 out]
            n216 = call "CC System Message.vi"("Message"=w371) -> ()  [unwired: 10 in, 1 out]
            n217 = Get Date/Time In Seconds() -> (seconds since 1Jan1904=w374:timestamp)
            n218 = Bundle By Name(cluster=w379, "Dither.index"=0, "Acq Settings"=w364, "timer"=w374, "Exposure"=w361, "target"=w366, "Target RA and DEC"=w365, "Script State"=w375) -> (w380:T24)
          }
          frame "script Acquire Wait Move" {
            # "Wait for telescope to finish moving."
            n219 = Unbundle By Name(w404) -> ("timer"=w399:timestamp, "Target RA and DEC"=w403:T10, "Exposure.Images"=w396:i32)
            n220 = call "CC Log Object.vi"("Action"=CC_enum_Current_Values_Action."Get Current Values") -> ("HK Channel out"=w411:refnum<class "HK Table.lvclass">)  [unwired: 8 in, 2 out]
            n221 = Get Date/Time In Seconds() -> (seconds since 1Jan1904=w401:timestamp)
            n222 = for {
              tunnel: w411 -> [w415]
              tunnel: string[] ["Telescope RA", "Telescope DEC", "Telescope Moving?", "Telescope Status"] -> [w414] mode=indexing
              tunnel: [w413] -> w409 mode=indexing
              n223 = call-dynamic "HK Read Value.vi"("Channel Name"=w414, "HK Channel in"=w415) -> ("Value"=w413:dbl)  [unwired: 4 in, 5 out]
            }
            n224 = Subtract(x=w401, y=w399) -> (x-y=w402:dbl)
            n225 = Less?(x=w402, y=180.0) -> (x < y?=w398:bool)
            n226 = Index Array(array=w409) -> (element #1=w406:dbl, element #2=w405:dbl, element #3=w408:dbl)  [unwired: 4 in, 1 out]
            n227 = Equal To 0?(x=w408) -> (x = 0?=w397:bool)
            n228 = case shown="True" w397 {
              tunnel: w404 -> [w416 w430]
              tunnel: [w417 w431] -> w407
              tunnel: w406 -> [_ w434]
              tunnel: w405 -> [_ w433]
              tunnel: w403 -> [_ w435]
              tunnel: w398 -> [w418 _]
              tunnel: w396 -> [_ w428]
              frame False {
                n229 = case shown="True" w418 {
                  tunnel: w416 -> [w421 w423]
                  tunnel: [w420 w423] -> w417
                  frame False {
                    n230 = call "CC System Message.vi"("Message"="Timeout waiting for telescope to reach position.") -> ()  [unwired: 10 in, 1 out]
                    n231 = Bundle By Name(cluster=w421, "Script State"="Script Error") -> (w420:T24)
                  }
                  frame True {
                  }
                }
              }
              frame True {
                # "Not moving"
                n232 = Bundle(cluster=w435, "RA"=w434, "DEC"=w433) -> (w432:T10)
                n233 = call "CC Script Check Telescope is Close Enough.vi"("Current Pos"=w432, "Target Pos"=w435) -> ("msg"=w424:string, "close enough"=w427:bool)  [unwired: 7 in, 1 out]
                n234 = case shown="True" w427 {
                  tunnel: w428 -> [_ w438]
                  tunnel: w424 -> [w436 _]
                  frame False {
                    n235 = call "CC System Message.vi"("Message"=w436) -> ()  [unwired: 10 in, 1 out]
                  }
                  frame True {
                    n236 = Format Into String(format string="Image 1 of %d.", w438) -> (resulting string=w437:string)  [unwired: 2 in, 1 out]
                    n237 = call "CC System Message.vi"("Message"=w437) -> ()  [unwired: 10 in, 1 out]
                  }
                }
                n238 = Select(t="script Read Detectors", s=w427, f="Script Error" ("Script State")) -> (s? t:f=w429:string)
                n239 = Bundle By Name(cluster=w430, "Script State"=w429) -> (w431:T24)
              }
            }
          }
          frame "script Read Detectors" {
            n240 = Unbundle By Name(w451) -> ("Exp Map"=w458:map{string, T6}, "Acq Settings.Exposure"=w457:string, "Cmd Qs.Detector Q"=w456:T2)
            n241 = Remove From Map(10:w457, 11:w458) -> (1:w442:T6)  [unwired: 2 out]
            n242 = Unbundle By Name(w442) -> ("Images"=w443:i32, "Name"=w446:string, "Mode"=w445:T7, "Integration Time"=w444:dbl)
            n243 = Bundle By Name(cluster=T26 {"Cmd"="Acquire Image", "Parameters"=variant} ("element"), "Parameters"=w442) -> (w454:T26)
            n244 = Enqueue Element(queue=w456, element=w454) -> ()  [unwired: 2 in, 3 out]
            n245 = Get Date/Time In Seconds() -> (seconds since 1Jan1904=w450:timestamp)
            n246 = Format Into String(format string="Detector exposure settings \"%s\" mode %s, integration time %f, collection %d images.", w446, w445, w444, w443) -> (resulting string=w440:string)  [unwired: 2 in, 1 out]
            n247 = Bundle By Name(cluster=w451, "timer"=w450, "Script State"="script Wait for Image", "Images Received"=FALSE) -> (w452:T24)
            n248 = call "CC System Message.vi"("Message"="Commanding Detetor to acquire images." ("format string")) -> ("error out"=w441:errorcluster)  [unwired: 10 in]
            n249 = call "CC System Message.vi"("error in (no error)"=w441, "Message"=w440) -> ()  [unwired: 9 in, 1 out]
          }
          frame "script Wait for Image" {
            # "Waiting for detector system to return images via script Q. State \"New Images\" sets the state so we can move on."
            n250 = Unbundle By Name(w462) -> ("timer"=w461:timestamp, "Images Received"=w466:bool, "Acq Settings"=w460:T13)
            n251 = Get Date/Time In Seconds() -> (seconds since 1Jan1904=w470:timestamp)
            n252 = Subtract(x=w470, y=w461) -> (x-y=w469:dbl)
            n253 = Greater?(x=w469, y=3660.0) -> (0:w467:bool)
            n254 = case shown="False" w467 {
              tunnel: w466 -> [w480 _]
              tunnel: w465 -> [w479 _]
              tunnel: [w477 "Script Error"] -> w464
              tunnel: w462 -> [w476 w481]
              tunnel: w460 -> [w475 _]
              tunnel: [w471 w481] -> w459
              frame False {
                n255 = Unbundle By Name(w475) -> ("Object"=w474:string, "Exposure"=w473:string, "Dithering"=w472:string)
                n256 = Select(t="Next Image", s=w480, f=w479) -> (s? t:f=w477:string)
                n257 = Bundle By Name(cluster=w476, "Obs.Object"=w474, "Obs.Detector Settings"=w473, "Obs.Dithering Type"=w472) -> (w471:T24)
              }
              frame True {
                # "time out. Report error and abort"
                n258 = call "CC System Message.vi"("Message"="Timeout waiting for detector to return images.") -> ()  [unwired: 10 in, 1 out]
              }
            }
            n259 = Bundle By Name(cluster=w459, "Script State"=w464) -> (w463:T24)
          }
          frame "Next Image" {
            n260 = Unbundle By Name(w494) -> ("Exposure.Images"=w486:i32, "Image idx"=w491:i32, "Data Q"=w493:refnum<queue>, "Total Images"=w492:i32)
            n261 = Increment(x=w492) -> (x+1=w485:i32)
            n262 = Decrement(x=w491) -> (x-1=w489:i32)
            n263 = call "CC Script Set Status Value.vi"("Value"=w485, "Ch Name"="Script Image Count", "Data Q"=w493) -> ()  [unwired: 8 in, 1 out]
            n264 = Greater Than 0?(x=w489) -> (x > 0?=w490:bool)
            n265 = case shown="True" w490 {
              tunnel: w489 -> [_ w504]
              tunnel: [w498 w504] -> w488
              tunnel: ["Next Dither" "script Read Detectors"] -> w487
              tunnel: w486 -> [w498 w502]
              tunnel: ["Images complete. Going to next dither." w501] -> w484
              frame False {
              }
              frame True {
                n266 = Subtract(x=w502, y=w504) -> (x-y=w503:i32)
                n267 = Increment(x=w503) -> (x+1=w500:i32)
                n268 = Format Into String(format string="Image %d of %d.", w500, w502) -> (resulting string=w501:string)  [unwired: 2 in, 1 out]
              }
            }
            n269 = Bundle By Name(cluster=w494, "Image idx"=w488, "Script State"=w487, "Total Images"=w485) -> (w496:T24)
            n270 = call "CC System Message.vi"("Message"=w484) -> ()  [unwired: 10 in, 1 out]
          }
          frame "Next Dither" {
            n271 = Unbundle By Name(w519) -> ("Dither"=w515:T36, "target"=w514:T8, "Cmd Qs.Telescope Q"=w520:T2, "Data Q"=w511:refnum<queue>)
            n272 = call "CC Script Next Dither.vi"("object"=w514, "Dither"=w515) -> ("Dither?"=w513:bool, "object"=w509:T8, "Dither out"=w510:T37, "Message"=w507:string)  [unwired: 5 in, 1 out]
            n273 = case shown="True" w513 {
              tunnel: w509 -> [_ w537]
              tunnel: w520 -> [_ w536]
              tunnel: ["Next Step" "script Acquire Wait Move" ("Script State")] -> w518
              tunnel: ["Image acquisition and dithering complete." ("format string") w529] -> w512
              tunnel: w510 -> [_ w533]
              tunnel: w511 -> [w522 w531]
              tunnel: w507 -> [_ w529]
              frame False {
                w521 = 0.0 ("Value")
                n274 = call "CC Script Set Status Value.vi"("Value"=w521, "Ch Name"="Script Dither Total", "Data Q"=w522) -> ()  [unwired: 8 in, 1 out]
                n275 = call "CC Script Set Status Value.vi"("Value"=w521, "Ch Name"="Script Dither Count", "Data Q"=w522) -> ()  [unwired: 8 in, 1 out]
              }
              frame True {
                n276 = Unbundle By Name(w533) -> ("index"=w534:i32)
                n277 = Bundle By Name(cluster=T26 {"Cmd"="Move", "Parameters"=variant} ("element"), "Parameters"=w537) -> (w539:T26)
                n278 = Increment(x=w534) -> (x+1=w532:i32)
                n279 = call "CC Script Set Status Value.vi"("Value"=w532, "Ch Name"="Script Dither Count", "Data Q"=w531) -> ()  [unwired: 8 in, 1 out]
                n280 = Enqueue Element(queue=w536, element=w539) -> (error out=w528:errorcluster)  [unwired: 2 in, 2 out]
                n281 = call "Stall Data Flow.vim"("value in"=w528, "milliseconds to wait"=u32 4000) -> ()  [unwired: 2 out]
              }
            }
            n282 = Unbundle By Name(w509) -> ("RA and DEC"=w508:T10)
            n283 = Get Date/Time In Seconds() -> (seconds since 1Jan1904=w516:timestamp)
            n284 = Bundle By Name(cluster=w519, "timer"=w516, "Target RA and DEC"=w508, "Dither"=w510, "Script State"=w518) -> (w517:T24)
            n285 = call "CC System Message.vi"("Message"=w512) -> ()  [unwired: 10 in, 1 out]
          }
          frame "script Telescope Move" {
            # "give telescope time to start\nmoving."
            n286 = Unbundle By Name(w543) -> ("Run Script"=w552:T4[], "step"=w551:i32, "Cmd Qs.Telescope Q"=w549:T2)
            n287 = Index Array(array=w552, index=w551) -> (element=w550:T4)
            n288 = Unbundle By Name(w550) -> ("Data"=w547:variant)
            n289 = Bundle By Name(cluster=T26 {"Cmd"="Move Focus", "Parameters"=variant} ("element"), "Parameters"=w547) -> (w546:T26)
            n290 = Enqueue Element(queue=w549, element=w546) -> (error out=w542:errorcluster)  [unwired: 2 in, 2 out]
            n291 = call "CC System Message.vi"("Message"="Script commanding telescope to move." ("format string")) -> ()  [unwired: 10 in, 1 out]
            n292 = call "Stall Data Flow.vim"("value in"=w542, "milliseconds to wait"=u32 2000) -> ()  [unwired: 2 out]
            n293 = Bundle By Name(cluster=w543, "Script State"="script Wait for Telescope Move") -> (w544:T24)
          }
          frame "script Telescope Home" {
            # "give telescope time to start\nmoving."
            n294 = Unbundle By Name(w556) -> ("Run Script"=w565:T4[], "step"=w564:i32, "Cmd Qs.Telescope Q"=w562:T2)
            n295 = Index Array(array=w565, index=w564) -> (element=w563:T4)
            n296 = Unbundle By Name(w563) -> ("Data"=w560:variant)
            n297 = Bundle By Name(cluster=T26 {"Cmd"="Home Focus", "Parameters"=variant} ("element"), "Parameters"=w560) -> (w559:T26)
            n298 = call "CC System Message.vi"("Message"="Script commanding telescope to home the focus." ("format string")) -> ()  [unwired: 10 in, 1 out]
            n299 = Enqueue Element(queue=w562, element=w559) -> (error out=w555:errorcluster)  [unwired: 2 in, 2 out]
            n300 = call "Stall Data Flow.vim"("value in"=w555, "milliseconds to wait"=u32 2000) -> ()  [unwired: 2 out]
            n301 = Bundle By Name(cluster=w556, "Script State"="script Wait for Telescope Move") -> (w557:T24)
          }
          frame "script Telescope RA DEC" {
            (unwired) CC_enum_Script_Action."Telescope RA DEC" ("Action")
            # "give telescope time to start\nmoving."
            n302 = Unbundle By Name(w575) -> ("Run Script"=w583:T4[], "step"=w582:i32, "Cmd Qs.Telescope Q"=w580:T2)
            n303 = Index Array(array=w583, index=w582) -> (element=w581:T4)
            n304 = Unbundle By Name(w581) -> ("Data"=w572:variant)
            n305 = Variant To Data(type=T10 {"RA"=0.0, "DEC"=0.0} ("RA and DEC"), Variant=w572) -> (data=w570:T10)  [unwired: 1 in, 1 out]
            n306 = Bundle By Name(cluster=T26 {"Cmd"="Move", "Parameters"=variant} ("element"), "Parameters"=w572) -> (w578:T26)
            n307 = call "CC Convert RA and DEC to HHMMSS.vi"("RA and DEC"=w570) -> ("DEC String"=w568:string, "RA String"=w567:string)  [unwired: 9 in]
            n308 = Enqueue Element(queue=w580, element=w578) -> (error out=w574:errorcluster)  [unwired: 2 in, 2 out]
            n309 = Format Into String(format string="Script commanding telescope to move to RA %s, DEC %s.", w567, w568) -> (resulting string=w566:string)  [unwired: 2 in, 1 out]
            n310 = call "CC System Message.vi"("Message"=w566) -> ()  [unwired: 10 in, 1 out]
            n311 = call "Stall Data Flow.vim"("value in"=w574, "milliseconds to wait"=u32 2000) -> ()  [unwired: 2 out]
            n312 = Bundle By Name(cluster=w575, "Script State"="script Wait for Telescope Move") -> (w576:T24)
          }
          frame "script Wait for Telescope Move" {
            n313 = call "CC Log Object.vi"("Action"=CC_enum_Current_Values_Action."Get Current Values") -> ("HK Channel out"=w590:refnum<class "HK Table.lvclass">)  [unwired: 8 in, 2 out]
            n314 = for {
              tunnel: w590 -> [w598]
              tunnel: string[] ["Telescope RA", "Telescope DEC", "Telescope Moving?", "Telescope Status"] -> [w597] mode=indexing
              tunnel: [w596] -> w588 mode=indexing
              n315 = call-dynamic "HK Read Value.vi"("Channel Name"=w597, "HK Channel in"=w598) -> ("Value"=w596:dbl)  [unwired: 4 in, 5 out]
            }
            n316 = Index Array(array=w588) -> (element #3=w587:dbl)  [unwired: 4 in, 3 out]
            n317 = Equal To 0?(x=w587) -> (x = 0?=w586:bool)
            n318 = case shown="False" w586 {
              tunnel: w584 -> [w594 w595]
              tunnel: [w592 w595] -> w585
              frame False {
                n319 = Bundle By Name(cluster=w594, "Script State"="Next Step") -> (w592:T24)
              }
              frame True {
              }
            }
          }
          frame "Ask User", "script Ask User" {
            n320 = Unbundle By Name(w599) -> ("Parameters"=w602:variant)
            n321 = Variant To Data(type="", Variant=w602) -> (data=w605:string, error out=w604:errorcluster)  [unwired: 1 in]
            n322 = case shown="No Error" w604 {
              tunnel: ["User Notification" ("Message") w608] -> w603
              tunnel: w602 -> [_ w610]
              frame No Error {
              }
              frame Error {
                n323 = call <vilib>:"Get Type Information.vi"("variant"=w610) -> ("name"=w609:string)  [unwired: 6 in, 4 out]
                n324 = Format Into String(format string="Software System Error in scripting. Ask User state parameter should be string but was not. Variant contents: %s", w609) -> (resulting string=w608:string)  [unwired: 2 in, 1 out]
              }
            }
            n325 = One Button Dialog(message=w605) -> ()  [unwired: 1 in, 1 out]
            n326 = Bundle By Name(cluster=w599, "Script State"="next step") -> (w600:T24)
            n327 = call "CC System Message.vi"("Message"=w603) -> ()  [unwired: 10 in, 1 out]
          }
          frame "next step" {
            n328 = Unbundle By Name(w615) -> ("step"=w619:i32, "Run Script"=w618:T4[], "paused"=w612:bool)
            n329 = Increment(x=w619) -> (x+1=w614:i32)
            n330 = Array Size(array=w618) -> (size(s)=w617:i32)
            n331 = Greater Or Equal?(x=w614, y=w617) -> (x >= y?=w616:bool)
            n332 = case shown="False" w616 {
              tunnel: w615 -> [w623 w629]
              tunnel: w614 -> [w622 _]
              tunnel: [w621 w630] -> w613
              tunnel: w612 -> [w620 _]
              frame False {
                n333 = case shown="False" w620 {
                  tunnel: w623 -> [w627 w628]
                  tunnel: w622 -> [w626 _]
                  tunnel: [w625 w628] -> w621
                  frame False {
                    n334 = Bundle By Name(cluster=w627, "step"=w626, "Script State"="execute step" ("event data")) -> (w625:T24)
                  }
                  frame True {
                  }
                }
              }
              frame True {
                n335 = Bundle By Name(cluster=w629, "Script State"="end script" ("event data")) -> (w630:T24)
              }
            }
          }
          frame "end script" {
            w635 = "" ("Step Name")
            n336 = Unbundle By Name(w643) -> ("Script Settings.Script Name"=w646:string, "Script Status Q"=w641:refnum<queue>, "Data Q"=w632:refnum<queue>)
            n337 = Get Date/Time In Seconds() -> (seconds since 1Jan1904=w634:timestamp)
            n338 = Format Into String(format string="Script %s finished", w646) -> (resulting string=w647:string)  [unwired: 2 in, 1 out]
            n339 = call "CC Script Send Script End Status.vi"("Data Q"=w632) -> ()  [unwired: 10 in, 1 out]
            n340 = Bundle By Name(cluster=T30 {"Time"=timestamp(0 s since 1904-01-01), "Running"=FALSE, "Step"=0, "Script Name"="", "Step Name"=""}, "Running"=FALSE, "Step"=0, "Step Name"=w635, "Script Name"=w635, "Time"=w634) -> (w633:T30)
            n341 = call "CC System Message.vi"("Message"=w647) -> ()  [unwired: 10 in, 1 out]
            n342 = Bundle By Name(cluster=w643, "Script Running"=FALSE, "Script State"="idle") -> (w644:T24)
            n343 = Bundle By Name(cluster=T28 {"Msg"="Status", "Data"=variant} ("element"), "Data"=w633) -> (w639:T28)
            n344 = Enqueue Element(queue=w641, element=w639) -> ()  [unwired: 2 in, 3 out]
          }
          frame "abort script" {
            n345 = Unbundle By Name(w651) -> ("Script Settings.Script Name"=w653:string, "Script Running"=w650:bool)
            n346 = case shown="False" w650 {
              tunnel: w653 -> [_ w660]
              tunnel: [w655 w659] -> w652
              tunnel: w651 -> [w655 w658]
              tunnel: ["Script Abort received but script not running" w656] -> w649
              frame False {
              }
              frame True {
                n347 = Format Into String(format string="Script %s aborted.", w660) -> (resulting string=w656:string)  [unwired: 2 in, 1 out]
                n348 = Bundle By Name(cluster=w658, "Script State"="end script") -> (w659:T24)
              }
            }
            n349 = call "CC System Message.vi"("Message"=w649) -> ()  [unwired: 10 in, 1 out]
          }
          frame "script error" {
            n350 = Unbundle By Name(w662) -> ("Data Q"=w665:refnum<queue>)
            n351 = call "CC Script Set Status Value.vi"("Value"=2.0, "Ch Name"="Script State", "Data Q"=w665) -> ()  [unwired: 8 in, 1 out]
            n352 = Bundle By Name(cluster=w662, "Script State"="abort script") -> (w666:T24)
          }
          frame "Shutdown" {
            n353 = Unbundle By Name(w670) -> ("Script Settings"=w669:T3)
            n354 = call "Rd Wr Script Defaults.vi"("Write? (F:Read)"=TRUE, "Script Settings"=w669) -> ()  [unwired: 8 in, 2 out]
          }
        }
      }
      event "Script Path": Value Change {
        n355 = event-data() -> ()  [unwired: 1 in, 6 out]
        n356 = Unbundle By Name(w677) -> ("state"=w676:refnum<user-event>)
        n357 = Generate User Event(user event=w676, event data cluster="init" ("event data")) -> ()  [unwired: 2 in, 2 out]
        n358 = Bundle By Name(cluster=w677, "Script Settings.Script Path"="Script Path") -> (w674:T24)
        n359 = Unbundle By Name(w674) -> ("Script Settings"=w673:T3)
        n360 = call "Rd Wr Script Defaults.vi"("Write? (F:Read)"=TRUE, "Script Settings"=w673) -> ()  [unwired: 8 in, 2 out]
      }
      event "Script": Shortcut Menu Activation? {
        n361 = event-data() -> ("CtlRef"=w687:refnum<vi>, "MenuRef"=w685:refnum<k9>, "Coords"=w686:T38)  [unwired: 1 in, 1 out]
        n362 = Unbundle By Name(w680) -> ("Script Settings.Script Path"=w679:path)
        n363 = call "CC Rd Wr Script.vi"("Script Path"=w679, "Action"=CC_Rd_Wr_Script_Action."List") -> ("Script List"=w682:string[])  [unwired: 4 in, 5 out]
        n364 = invoke class="MCListbox (strict)" method="Point To Row Column"(reference=w687, "Point"=w686) -> ()  [unwired: 5 in, 7 out]
        n365 = for {
          tunnel: w682 -> [w690] mode=indexing
          tunnel: [w689] -> w681 mode=indexing
          n366 = Format Into String(format string="Insert|%s", w690) -> (resulting string=w689:string)  [unwired: 2 in, 1 out]
        }
        n367 = Insert Menu Items(5:"Insert" ("menu tag"), 7:w681, 8:w682, 9:w685) -> ()  [unwired: 2 in, 3 out]
        n368 = event-data("Discard?"=FALSE) -> ()  [unwired: 1 in, 1 out]
      }
      event "Script": Shortcut Menu Selection (User) {
        n369 = event-data() -> ("ItemTag"=w699:string, "CtlRef"=w704:refnum<vi>, "Coords"=w703:T38)  [unwired: 1 in, 5 out]
        n370 = Unbundle By Name(w695) -> ("state"=w693:refnum<user-event>, "Script"=w700:T4[], "Script Settings.Script Path"=w692:path)
        n371 = invoke class="MCListbox (strict)" method="Point To Row Column"(reference=w704, "Point"=w703) -> ("CellPosition"=w702:T39)  [unwired: 5 in, 6 out]
        n372 = Match Pattern(string=w699, regular expression="|") -> (before substring=w697:string, after substring=w696:string)  [unwired: 1 in, 2 out]
        n373 = Unbundle By Name(w702) -> ("Row"=w701:i32)
        n374 = case shown="\"Insert\"" w697 {
          tunnel: w701 -> [_ w708 w710 w729]
          tunnel: w700 -> [_ w709 _ w730]
          tunnel: w696 -> [_ _ _ w733]
          tunnel: w695 -> [w705 w706 w711 w724]
          tunnel: [w705 w706 w715 w722] -> w694
          tunnel: w693 -> [_ _ _ w721]
          tunnel: w692 -> [_ _ _ w718]
          frame "False", Default {
          }
          frame "Execute Step" {
            n375 = Index Array(array=w709, index=w708) -> (element=w707:T4)
            n376 = call "CC Script Execute Step.vi"("Script Step"=w707) -> ()  [unwired: 10 in, 1 out]
          }
          frame "Continue From This Step" {
            n377 = Unbundle By Name(w711) -> ("Script Settings.Script Name"=w713:string)
            n378 = Bundle By Name(cluster=w711, "step"=w710, "Script Running"=TRUE, "Script State"="execute step" ("event data")) -> (w715:T24)
            n379 = Format Into String(format string="Continuing Script \"%s\" from step %d" ("Message"), w713, w710) -> (resulting string=w712:string)  [unwired: 2 in, 1 out]
            n380 = call "CC System Message.vi"("Message"=w712) -> ()  [unwired: 10 in, 1 out]
          }
          frame "Insert" {
            n381 = Bundle By Name(cluster=T29 {"Name"="", "Script"=[]} ("Script"), "Name"=w733) -> (w732:T29)
            n382 = Increment(x=w729) -> (x+1=w719:i32)
            n383 = Generate User Event(user event=w721, event data cluster="show script" ("event data")) -> ()  [unwired: 2 in, 2 out]
            n384 = Split 1D Array(array=w730, index=w719) -> (first subarray=w726:T4[], second subarray=w727:T4[])
            n385 = call "CC Rd Wr Script.vi"("Script Path"=w718, "Action"=CC_Rd_Wr_Script_Action."Read", "Script"=w732) -> ("Script"=w728:T29)  [unwired: 3 in, 5 out]
            n386 = Unbundle By Name(w728) -> ("Script"=w725:T4[])
            n387 = Build Array (concatenate)(w726, w725, w727) -> (w723:T4[])
            n388 = Bundle By Name(cluster=w724, "Script"=w723) -> (w722:T24)
          }
        }
      }
      event "Script": Value Change {
        n389 = event-data() -> ("NewVal"=w739:string)  [unwired: 1 in]
        n390 = Unbundle By Name(w737) -> ("state"=w736:refnum<user-event>)
        n391 = Generate User Event(user event=w736, event data cluster="load script" ("event data")) -> ()  [unwired: 2 in, 2 out]
        n392 = Bundle By Name(cluster=w737, "Script Settings.Script Name"=w739) -> (w738:T24)
      }
      event "Edit Script", "New Script": Value Change {
        n393 = event-data() -> ()  [unwired: 1 in, 6 out]
        n394 = Unbundle By Name(w742) -> ("script edit ref"=w741:refnum<vi>)
        n395 = property class="VI Interface Type 0"(reference=w741) -> ("FP.State"=w740:T40)  [unwired: 1 in, 2 out]
        n396 = Select(t="", s="New Script", f="Script") -> (s? t:f=w744:string)
        n397 = case shown="\"Invalid\", Default" w740 {
          tunnel: w744 -> [w752 _]
          tunnel: [w751 w759] -> w743
          tunnel: w742 -> [w750 w759]
          tunnel: w741 -> [_ w761]
          frame "Invalid", Default {
            n398 = vi-ref "CC Create Script.vi"() -> (w757:refnum<vi>)
            n399 = property class="VI (strict)"(reference=w757) -> (error out=w758:errorcluster, "Path"=w756:path)  [unwired: 1 in, 1 out]
            n400 = Open VI Reference(type specifier VI Refnum (for type only)=w757, vi path=w756, options=128, error in (no error)=w758) -> (vi reference=w755:refnum<vi>, error out=w753:errorcluster)  [unwired: 2 in]
            n401 = call-by-ref "Start Asynchronous Call"(reference=w755, error in=w753, "script name in"=w752) -> (reference out=w749:refnum<vi>)  [unwired: 10 in, 2 out]
            n402 = invoke class="VI Interface Type 4" method="FP.Open"(reference=w749, "Activate"=TRUE ("Activate?")) -> ()  [unwired: 3 in, 5 out]
            n403 = Bundle By Name(cluster=w750, "script edit ref"=w749) -> (w751:T24)
          }
          frame "Standard" {
            n404 = property class="VI Interface Type 0"(reference=w761, "Front Panel.IsFrontmost"=TRUE ("Front Panel Window:Is Frontmost")) -> ()  [unwired: 1 in, 2 out]
          }
        }
      }
      event "Run Script": Value Change {
        n405 = event-data() -> ()  [unwired: 1 in, 6 out]
        n406 = Unbundle By Name(w764) -> ("state"=w763:refnum<user-event>)
        n407 = Generate User Event(user event=w763, event data cluster="start script" ("event data")) -> ()  [unwired: 2 in, 2 out]
      }
      event "Stop Script": Value Change {
        n408 = event-data() -> ()  [unwired: 1 in, 6 out]
        n409 = Unbundle By Name(w767) -> ("state"=w766:refnum<user-event>)
        n410 = Generate User Event(user event=w766, event data cluster="abort script" ("event data")) -> ()  [unwired: 2 in, 2 out]
      }
      event "Close": Value Change {
        n411 = event-data() -> ()  [unwired: 1 in, 2 out]
        n412 = Unbundle By Name(w770) -> ("state"=w769:refnum<user-event>)
        n413 = Generate User Event(user event=w769, event data cluster="shutdown" ("event data")) -> ()  [unwired: 2 in, 2 out]
      }
    }
  }
